vi "JO4MCrossover.vi"(8 "error in (no error)":errorcluster, 9 "Parent 2":T1, 10 "Parent 1":T1, 11 "OSSP_Problem in":refnum<class "OSSP_Problem.lvclass">) -> (0 "error out":errorcluster, 1 "Child 2":T1, 2 "Child 1":T1, 3 "OSSP_Problem out":refnum<class "OSSP_Problem.lvclass">)   [LabVIEW 2013, in "GA.lvclass"]
uses:
  GA.lvclass
  Controls/Solution_GA.ctl
  OSSP_Problem.lvclass
  OSSP_Problem.lvclass/OSSP_Problem.ctl
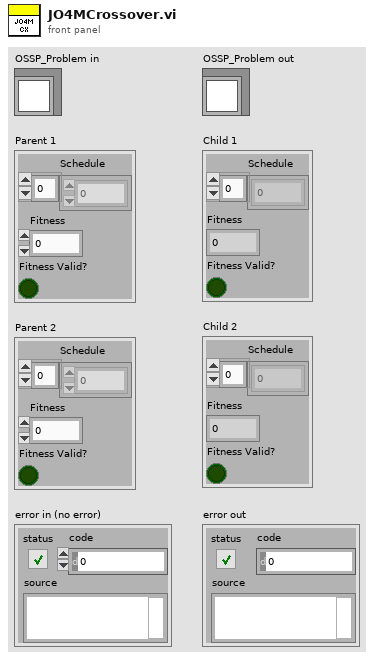
[diagram p1: front panel]
types:
  T1 = typedef "Solution_GA.ctl" = cluster{"Schedule":u16[], "Fitness":u16, "Fitness Valid?":bool}
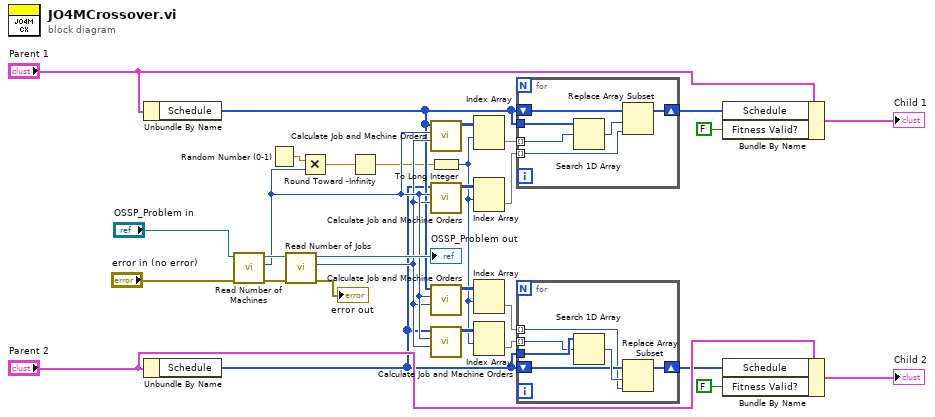
[diagram p0: block diagram]
diagram:
  n1 = Unbundle By Name("Parent 1") -> ("Schedule"=w8:u16[])
  n2 = Unbundle By Name("Parent 2") -> ("Schedule"=w4:u16[])
  n3 = call "Read Number of Machines.vi"("error in (no error)"="error in (no error)", "OSSP_Problem in"="OSSP_Problem in") -> ("error out"=w18:errorcluster, "Number of Machines"=w16:i32, "OSSP_Problem out"=w20:refnum<class "OSSP_Problem.lvclass">)  [unwired: 7 in]
  n4 = Random Number (0-1)() -> (number: 0 to 1=w24:dbl)
  n5 = call "Read Number of Jobs.vi"("error in (no error)"=w18, "OSSP_Problem in"=w20) -> ("error out"=→"error out":errorcluster, "Number of Jobs"=w15:i32, "OSSP_Problem out"=→"OSSP_Problem out":refnum<class "OSSP_Problem.lvclass">)  [unwired: 7 in]
  n6 = Multiply(x=w24, y=w16) -> (x*y=w23:dbl)
  n7 = Round Toward -Infinity(1:w23) -> (0:w2:dbl)
  n8 = call "Calculate Job and Machine Orders.vi"("Number of Jobs"=w15, "Number of Machines"=w16, "Schedule"=w8) -> ("JO4M"=w14:u16[][])  [unwired: 7 in, 1 out]
  n9 = To Long Integer(number=w2) -> (32bit integer=w1:i32)
  n10 = call "Calculate Job and Machine Orders.vi"("Number of Jobs"=w15, "Number of Machines"=w16, "Schedule"=w4) -> ("JO4M"=w12:u16[][])  [unwired: 7 in, 1 out]
  n11 = call "Calculate Job and Machine Orders.vi"("Number of Jobs"=w15, "Number of Machines"=w16, "Schedule"=w8) -> ("JO4M"=w13:u16[][])  [unwired: 7 in, 1 out]
  n12 = call "Calculate Job and Machine Orders.vi"("Number of Jobs"=w15, "Number of Machines"=w16, "Schedule"=w4) -> ("JO4M"=w11:u16[][])  [unwired: 7 in, 1 out]
  n13 = Index Array(array=w14, index (row)=w1) -> (element=w10:u16[])  [unwired: 1 in]
  n14 = Index Array(array=w12, index (row)=w1) -> (element=w9:u16[])  [unwired: 1 in]
  n15 = Index Array(array=w13, index (row)=w1) -> (element=w6:u16[])  [unwired: 1 in]
  n16 = Index Array(array=w11, index (row)=w1) -> (element=w5:u16[])  [unwired: 1 in]
  n17 = for {
    tunnel: w8 -> [w31]
    tunnel: w10 -> [w36] mode=indexing
    tunnel: w9 -> [w34] mode=indexing
    shift-right: [w32] -> w7
    shift-left: w8 -> [w33]
    n18 = Search 1D Array(1D array=w31, element=w36) -> (index of element=w35:i32)  [unwired: 1 in]
    n19 = Replace Array Subset(array=w33, new element=w34, index=w35) -> (w32:u16[])
  }
  n20 = for {
    tunnel: w4 -> [w39]
    tunnel: w6 -> [w37] mode=indexing
    tunnel: w5 -> [w38] mode=indexing
    shift-right: [w40] -> w3
    shift-left: w4 -> [w41]
    n21 = Search 1D Array(1D array=w39, element=w38) -> (index of element=w42:i32)  [unwired: 1 in]
    n22 = Replace Array Subset(array=w41, new element=w37, index=w42) -> (w40:u16[])
  }
  n23 = Bundle By Name(cluster="Parent 1", "Schedule"=w7, "Fitness Valid?"=FALSE) -> (→"Child 1":T1)
  n24 = Bundle By Name(cluster="Parent 2", "Schedule"=w3, "Fitness Valid?"=FALSE) -> (→"Child 2":T1)
